vi "Receive.vi"(8 "error in (no error)":errorcluster, 10 "Transfer Group in":refnum<class "Transfer Group.lvclass">, 11 "UDPlog Transceiver in":refnum<class "UDPlog Transceiver.lvclass">) -> (0 "error out":errorcluster, 2 "Transfer Group out":refnum<class "Transfer Group.lvclass">, 3 "UDPlog Transceiver out":refnum<class "UDPlog Transceiver.lvclass">)   [LabVIEW 2023, in "UDPlog.lvlib" / "UDPlog Transceiver.lvclass"]
uses:
  UDPlog Transceiver.lvclass
  Users/Public/Documents/National Instruments/NI VeriStand 2023/Custom Devices/Data Sharing Framework/Linux_x64/DSF Core.lvlibp/Classes/Transfer Group/Transfer Group.lvclass
  UDPlog Transceiver.lvclass/UDPlog Transceiver.ctl
  Read Datagram.vi
  <vilib>/Utility/error.llb/Clear Errors.vi
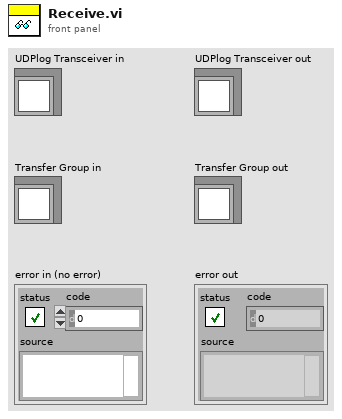
[diagram p1: front panel]
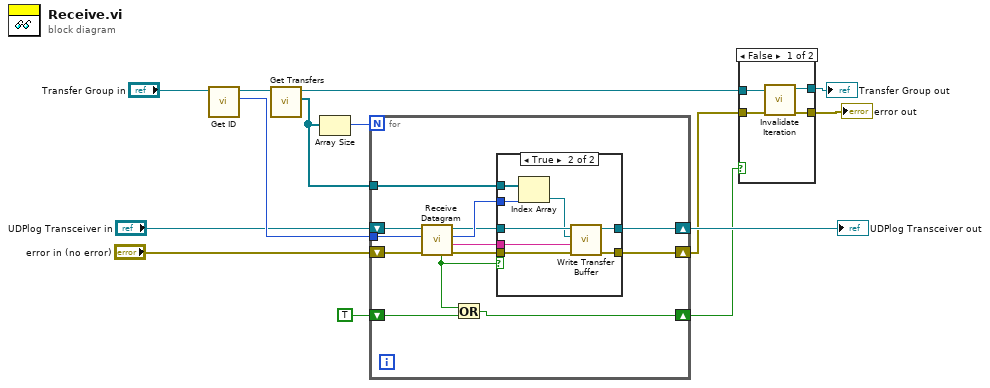
[diagram p0: block diagram]
diagram:
  n1 = call "Get ID.vi"("Transfer Group in"="Transfer Group in") -> ("id"=w3:i32, "Transfer Group out"=w14:refnum<class "Transfer Group.lvclass">)  [unwired: 9 in]
  n2 = call "Get Transfers.vi"("Transfer Group in"=w14) -> ("Transfers"=w2:refnum<class "Transfer.lvclass">[], "Transfer Group out"=w13:refnum<class "Transfer Group.lvclass">)  [unwired: 9 in]
  n3 = Array Size(array=w2) -> (size(s)=w9:i32)
  n4 = for {
    N: w9 -> [_]
    shift-right: [w17] -> w8
    shift-left: "UDPlog Transceiver in" -> [w27]
    shift-right: [w16] -> w6
    shift-left: "error in (no error)" -> [w25]
    shift-right: [w18] -> w4
    shift-left: TRUE -> [w19]
    tunnel: w3 -> [w26]
    tunnel: w2 -> [w15]
    n5 = call "Receive Datagram.vi"("error in (no error)"=w25, "transfer group id"=w26, "UDPlog Transceiver in"=w27) -> ("error out"=w24:errorcluster, "transfer data"=w21:string, "transfer id"=w23:i32, "UDPlog Transceiver out"=w22:refnum<class "UDPlog Transceiver.lvclass">, "valid"=w20:bool)  [unwired: 4 in]
    n6 = Or(x=w20, y=w19) -> (x .or. y?=w18:bool)
    n7 = case shown="True" w20 {
      tunnel: w24 -> [w28 w37]
      tunnel: w23 -> [_ w32]
      tunnel: w22 -> [w29 w35]
      tunnel: w21 -> [_ w36]
      tunnel: [w29 w33] -> w17
      tunnel: [w28 w34] -> w16
      tunnel: w15 -> [_ w31]
      frame False {
      }
      frame True {
        n8 = Index Array(array=w31, index=w32) -> (element=w30:refnum<class "Transfer.lvclass">)
        n9 = call "Write Transfer Buffer.vi"("error in (no error)"=w37, "data"=w36, "Transfer"=w30, "UDPlog Transceiver in"=w35) -> ("error out"=w34:errorcluster, "UDPlog Transceiver out"=w33:refnum<class "UDPlog Transceiver.lvclass">)  [unwired: 6 in]
      }
    }
  }
  "UDPlog Transceiver out" <- w8
  n10 = case shown="False" w4 {
    tunnel: w13 -> [w41 w43]
    tunnel: [w40 w43] -> w11
    tunnel: [w39 w42] -> w10
    tunnel: w6 -> [w38 w42]
    frame False {
      n11 = call "Invalidate Iteration.vi"("error in (no error)"=w38, "Transfer Group in"=w41) -> ("error out"=w39:errorcluster, "Transfer Group out"=w40:refnum<class "Transfer Group.lvclass">)  [unwired: 8 in]
    }
    frame True {
    }
  }
  "error out" <- w10
  "Transfer Group out" <- w11
